vi "Update TXT File.vi"(6 "Data Point":dbl, 8 "error in":errorcluster, 11 "Path":path) -> (0 "error out":errorcluster)   [LabVIEW 2009]
doc: "This sub VI is called by the TXT report class.\n\nAAL 9/09"
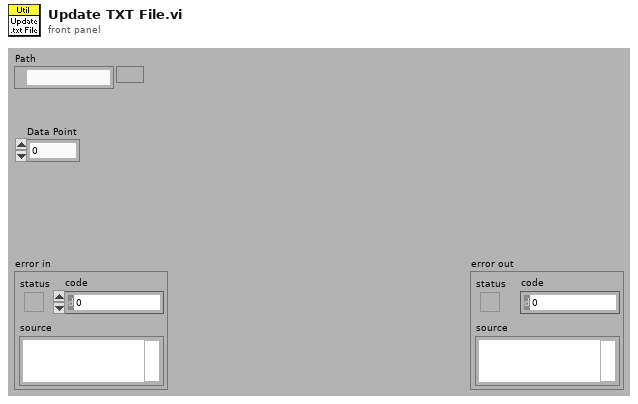
[diagram p1: front panel]
types:
  T1 = enum16{"open", "replace", "create", "open or create", "replace or create", "replace or create with confirmation"}
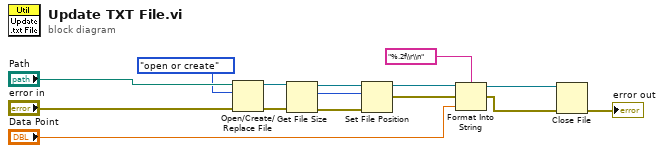
[diagram p0: block diagram]
diagram:
  n1 = Open/Create/Replace File(file path (use dialog)="Path", error in="error in", operation (0:open)=T1."open or create") -> (refnum out=w6:refnum<file>, error out=w7:errorcluster)  [unwired: 4 out]
  n2 = Get File Size(file=w6, error in=w7) -> (refnum out=w3:refnum<file>, size (in bytes)=w4:i64, 0:w5:errorcluster)
  n3 = Set File Position(offset (in bytes) (0)=w4, refnum=w3, error in=w5) -> (refnum out=w2:refnum<file>, error out=w1:errorcluster)  [unwired: 1 in]
  n4 = Format Into String(format string="%.2f\\r\\n", initial string=w2, error in=w1, "Data Point") -> (resulting string=w12:refnum<file>, error out=w11:errorcluster)
  n5 = Close File(refnum=w12, error in=w11) -> (error out=→"error out":errorcluster)  [unwired: 1 out]
